vi "PV ActiveLine Data.vi"(8 "error in (no error)":errorcluster, 9 "PV ActiveLine-Cluster":T1={"Parameter"=enum." Pressure  [mbar] (740)", "Parameter\nread only<->describe"=FALSE, "Correction facktor\n(0,20 - 9,90) "=1.0, "Pressure set point (mbar)\n0 ==> ur (p<1,0e-4 mbar)\n1 - 2050 mbar"=0} {"Pressure set point (mbar)\n0 ==> ur (p<1,0e-4 mbar)\n1 - 2050 mbar" min=0 max=2050 step=1; "Correction facktor\n(0,20 - 9,90)" min=0.2 max=9.9 step=0.01 format="%.2f"}, 10 "Adress of unit":u16=10 max=999 step=1, 11 "VISA session":refnum<visa-resource-name>) -> (0 "error out":errorcluster, 2 "response (data)":string, 3 "dup VISA session":refnum<visa-resource-name>)   [LabVIEW 2021, in "Pfeiffer Vacuum.lvlib"]
doc: "There are 5 parameters available, only one of which can be enabled at a time. \n\n0 - Pressure [mbar] (default) (740)\n1 - Correction factor sensor 1..6 (742)\n2 - Actual error code (read only) (303)\n3 - Software version Transmitter (read only) (312)\n4 - Unit type Transmitter (read only) (349)\n\nNote: The controls right of this one will set the appropriate values for the selected parameter. Any settings for an parameter that is not selected will be ignored. If a value is out of range, it will be changed to either the upper or the lower limit of the range."
uses:
  <instrlib>/Pfeiffer Vacuum/Pfeiffer Vacuum.lvlib
  <instrlib>/Pfeiffer Vacuum/Public/ActiveLine/PV ActiveLine - Cluster.ctl
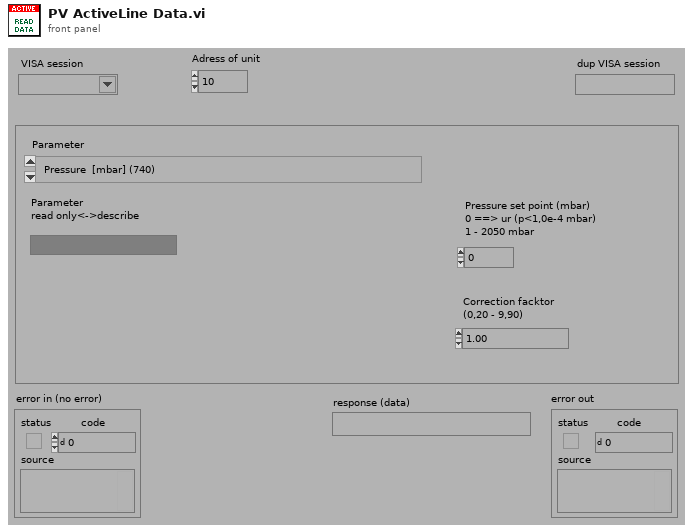
[diagram p1: front panel]
types:
  T1 = typedef "Pfeiffer Vacuum.lvlib/PV ActiveLine - Cluster.ctl" = cluster{"Parameter":enum16{" Pressure  [mbar] (740)", " Correction factor sensor (742)", " Actual error code (read only) (303)", " Software version Transmitter (read only) (312)", " Unit type Transmitter (read only) (349)"}, "Parameter\nread only<->describe":bool, "Correction facktor\n(0,20 - 9,90) ":sgl, "Pressure set point (mbar)\n0 ==> ur (p<1,0e-4 mbar)\n1 - 2050 mbar":i16}
  T2 = enum16{" Pressure  [mbar] (740)", " Correction factor sensor (742)", " Actual error code (read only) (303)", " Software version Transmitter (read only) (312)", " Unit type Transmitter (read only) (349)"}
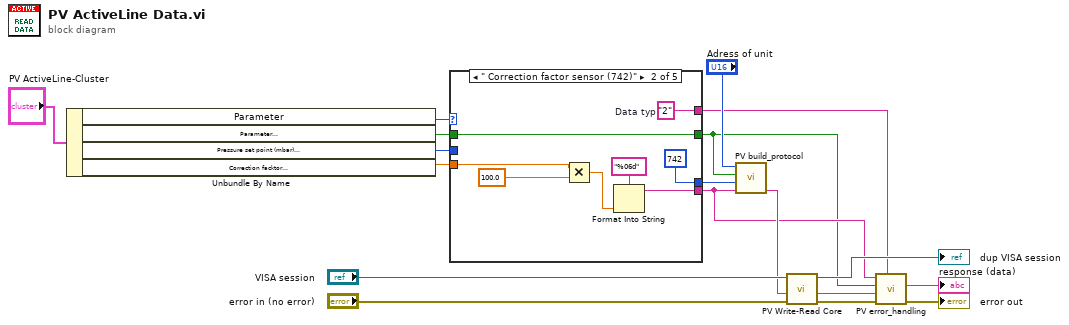
[diagram p0: block diagram]
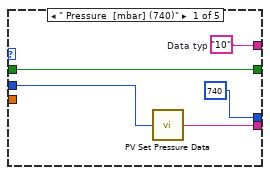
[diagram p2: hidden frame]
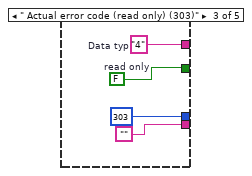
[diagram p3: hidden frame]
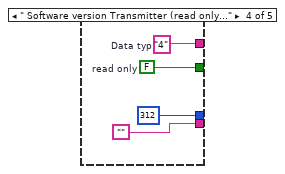
[diagram p4: hidden frame]
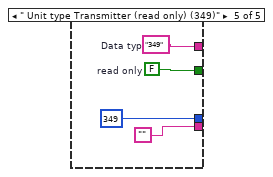
[diagram p5: hidden frame]
diagram:
  n1 = Unbundle By Name("PV ActiveLine-Cluster") -> ("Parameter"=w16:T2, "Parameter\nread only<->describe"=w15:bool, "Pressure set point (mbar)\n0 ==> ur (p<1,0e-4 mbar)\n1 - 2050 mbar"=w13:i16, "Correction facktor\n(0,20 - 9,90)"=w2:sgl)
  n2 = case shown="\" Correction factor sensor (742)\"" w16 {
    tunnel: [u16 740 ("Parameter-number") u16 742 ("Parameter-number") u16 303 ("Parameter-number") u16 312 ("Parameter-number") u16 349 ("Parameter-number")] -> w17
    tunnel: [w21 w24 "" "" ""] -> w5
    tunnel: [w22 w30 w34 w37 w43] -> w4
    tunnel: w15 -> [w22 w30 _ _ _]
    tunnel: w13 -> [w20 _ _ _ _]
    tunnel: w2 -> [_ w26 _ _ _]
    tunnel: [w19 w29 w32 w36 w40] -> w6
    frame " Pressure  [mbar] (740)" {
      w19 = "10"  # Data typ
      n3 = call <instrlib>:"PV Set Pressure Data.vi"("Pressure (mbar)\n0 ==> ur (<1,0e-4mbar)\n1 - 2050 mbar"=w20) -> ("Output"=w21:string)
    }
    frame " Correction factor sensor (742)" {
      w29 = "2"  # Data typ
      n4 = Multiply(x=w26, y=100.0) -> (x*y=w25:dbl)
      n5 = Format Into String(format string="%06d" ("Format-String"), w25) -> (resulting string=w24:string)  [unwired: 2 in, 1 out]
    }
    frame " Actual error code (read only) (303)" {
      w32 = "4"  # Data typ
      w34 = FALSE  # read only
    }
    frame " Software version Transmitter (read only) (312)" {
      w36 = "4"  # Data typ
      w37 = FALSE  # read only
    }
    frame " Unit type Transmitter (read only) (349)" {
      w40 = "349"  # Data typ
      w43 = FALSE  # read only
    }
  }
  n6 = call <instrlib>:"PV build_protocol.vi"("Data"=w5, "Parameter-number"=w17, "parameter\nread<->describe"=w4, "Adress"="Adress of unit") -> ("output"=w10:string)  [unwired: 3 in]
  n7 = call <instrlib>:"PV Write-Read Core.vi"("error in"="error in (no error)", "Write data in"=w10, "VISA session"="VISA session") -> ("error out"=w7:errorcluster, "response (data) out"=w8:string, "dup VISA session"=→"dup VISA session":refnum<visa-resource-name>)  [unwired: 2 in]
  n8 = call <instrlib>:"PV error_handling.vi"("Data Typ in"=w6, "error in"=w7, "response (data) in"=w8, "Parameter\nread only<->describe"=w4, "data in"=w5) -> ("error out"=→"error out":errorcluster, "Data out"=→"response (data)":string)  [unwired: 4 in, 1 out]
